vi "AnalogOutputs.vi"() -> ()   [LabVIEW 2016]
uses:
  controls/Enum.ctl
  <vilib>/rvi/errors/niLvFpgaAdjustHostInterfaceError.vi
  <vilib>/Utility/error.llb/Error Cluster From Error Code.vi
  controls/FPGAVIreferenceTypeDefScanEngine.ctl
  <vilib>/rvi/interface/nirviReadWriteControl/nirviReadWriteControl.xnode
  FPGA Bitfiles/lbniAFMControlle_scanControl_controllerFPGAPX_N4i+37z1gG8.lvbitx
  NiFpgaLv.dll
panel:
  in  "AO5.Activate":bool=TRUE
  in  "AO6.Activate":bool=TRUE
  in  "AO7.Activate":bool=TRUE
  in  "AO7":dbl(slide) caption="Bias" scale=-10.0..10.0
  in  "AO6":dbl(slide) caption="Bias" scale=-10.0..10.0
  in  "AO5":dbl(slide) caption="Bias" scale=-10.0..10.0
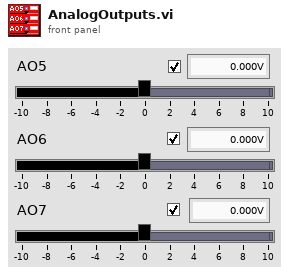
[diagram p1: front panel]
types:
  T1 = typedef "Enum.ctl" = enum16{"Init", "Read", "Write"}
  T2 = typedef "FPGAVIreferenceTypeDefScanEngine.ctl" = refnum<k20>
  T3 = enum8{"Enabled", "Disabled", "Disabled and Grayed Out"}
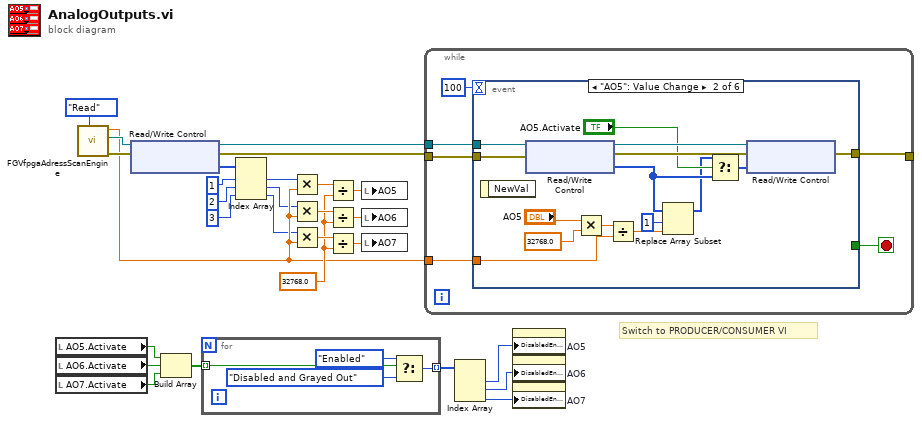
[diagram p0: block diagram]
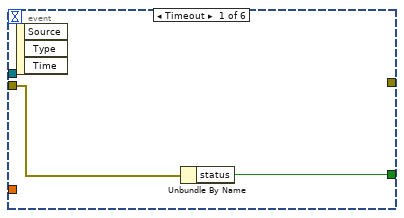
[diagram p2: hidden frame]
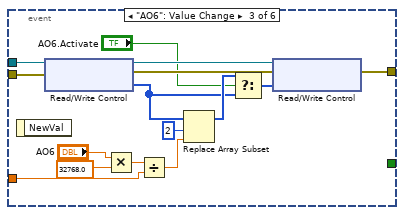
[diagram p3: hidden frame]
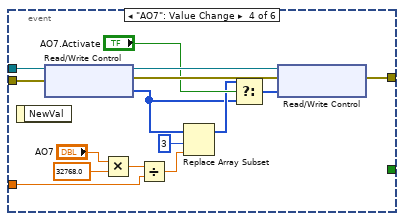
[diagram p4: hidden frame]
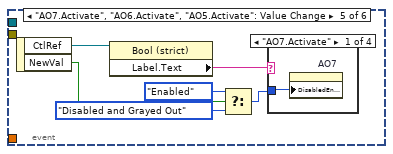
[diagram p5: hidden frame]
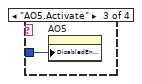
[diagram p7: hidden frame]
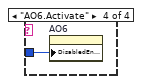
[diagram p8: hidden frame]
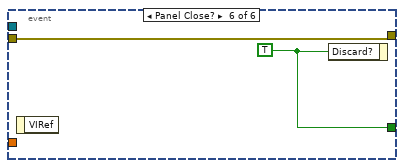
[diagram p9: hidden frame]
diagram:
  w5 = 32768.0 ("index")
  # "Switch to PRODUCER/CONSUMER VI"
  n1 = local read "AO5.Activate"() -> (w20:bool)
  n2 = local read "AO6.Activate"() -> (w19:bool)
  n3 = local read "AO7.Activate"() -> (w18:bool)
  n4 = call "FGVfpgaAdressScanEngine.vi"("Enum"=Enum."Read") -> ("error out"=w23:errorcluster, "FPGA.SEout"=w28:T2, "voltageRange(+/-)Out"=w4:dbl)  [unwired: 6 in, 2 out]
  n5 = xnode "Read/Write Control"("FPGA VI Reference In"=w28, "error in"=w23) -> ("FPGA VI Reference Out"=w10:T2, "error out"=w9:errorcluster, "aio.o.outputs"=w24:i16[])
  n6 = Build Array(w20, w19, w18) -> (w17:bool[])
  n7 = for {
    tunnel: w17 -> [w30] mode=indexing
    tunnel: [w29] -> w16 mode=indexing
    n8 = Select(t=T3."Enabled" ("Disabled"), s=w30, f=T3."Disabled and Grayed Out" ("Disabled")) -> (s? t:f=w29:T3)
  }
  n9 = Index Array(array=w24, index #1=1 ("index"), index #2=2 ("index"), index #3=3 ("index")) -> (element #1=w3:i16, element #2=w2:i16, element #3=w1:i16)
  n10 = Multiply(x=w3, y=w4) -> (x*y=w26:dbl)
  n11 = Multiply(x=w2, y=w4) -> (x*y=w22:dbl)
  n12 = Multiply(x=w1, y=w4) -> (x*y=w21:dbl)
  n13 = Divide(x=w26, y=w5) -> (x/y=w6:dbl)
  n14 = Divide(x=w22, y=w5) -> (x/y=w7:dbl)
  n15 = Divide(x=w21, y=w5) -> (x/y=w8:dbl)
  n16 = local write "AO5"(w6) -> ()
  n17 = local write "AO6"(w7) -> ()
  n18 = local write "AO7"(w8) -> ()
  n19 = while {
    tunnel: w4 -> [w35]
    tunnel: w9 -> [w33]
    tunnel: [w34] -> _
    tunnel: w10 -> [w36]
    stop <- w38 stop-if-true
    n20 = event shown="[1] \"AO5\": Value Change" {
      selector: _ -> [_ _ _ _ _ _]
      dyn-events: _ -> [_ _ _ _ _ _]
      timeout: 100 -> [_ _ _ _ _ _]
      tunnel: [w39 _ _ _ _ w96] -> w38
      tunnel: w36 -> [_ w48 w69 w83 _ _]
      tunnel: w35 -> [_ w46 w63 w78 _ _]
      tunnel: [_ w49 w66 w80 _ w95] -> w34
      tunnel: w33 -> [w40 w47 w67 w81 _ w95]
      event Timeout {
        n21 = event-data() -> ()  [unwired: 1 in, 3 out]
        n22 = Unbundle By Name(w40) -> ("status"=w39:bool)
      }
      event "AO5": Value Change {
        n23 = event-data() -> ()  [unwired: 1 in, 1 out]
        n24 = xnode "Read/Write Control"("FPGA VI Reference In"=w48, "error in"=w47) -> ("FPGA VI Reference Out"=w55:T2, "error out"=w50:errorcluster, "aio.o.outputs"=w43:i16[])
        n25 = Multiply(x="AO5", y=32768.0 ("index")) -> (x*y=w52:dbl)
        n26 = Divide(x=w52, y=w46) -> (x/y=w51:dbl)
        n27 = Replace Array Subset(array=w43, new element=w51, index=1) -> (w42:i16[])
        n28 = Select(t=w42, s="AO5.Activate", f=w43) -> (s? t:f=w41:i16[])
        n29 = xnode "Read/Write Control"("FPGA VI Reference In"=w55, "error in"=w50, "aio.o.outputs"=w41) -> ("error out"=w49:errorcluster)  [unwired: 1 out]
      }
      event "AO6": Value Change {
        n30 = event-data() -> ()  [unwired: 1 in, 1 out]
        n31 = xnode "Read/Write Control"("FPGA VI Reference In"=w69, "error in"=w67) -> ("FPGA VI Reference Out"=w68:T2, "error out"=w65:errorcluster, "aio.o.outputs"=w57:i16[])
        n32 = Multiply(x="AO6", y=32768.0 ("index")) -> (x*y=w60:dbl)
        n33 = Divide(x=w60, y=w63) -> (x/y=w64:dbl)
        n34 = Replace Array Subset(array=w57, new element=w64, index=2) -> (w59:i16[])
        n35 = Select(t=w59, s="AO6.Activate", f=w57) -> (s? t:f=w58:i16[])
        n36 = xnode "Read/Write Control"("FPGA VI Reference In"=w68, "error in"=w65, "aio.o.outputs"=w58) -> ("error out"=w66:errorcluster)  [unwired: 1 out]
      }
      event "AO7": Value Change {
        n37 = event-data() -> ()  [unwired: 1 in, 1 out]
        n38 = xnode "Read/Write Control"("FPGA VI Reference In"=w83, "error in"=w81) -> ("FPGA VI Reference Out"=w82:T2, "error out"=w85:errorcluster, "aio.o.outputs"=w72:i16[])
        n39 = Multiply(x="AO7", y=32768.0 ("index")) -> (x*y=w75:dbl)
        n40 = Divide(x=w75, y=w78) -> (x/y=w79:dbl)
        n41 = Replace Array Subset(array=w72, new element=w79, index=3) -> (w73:i16[])
        n42 = Select(t=w73, s="AO7.Activate", f=w72) -> (s? t:f=w71:i16[])
        n43 = xnode "Read/Write Control"("FPGA VI Reference In"=w82, "error in"=w85, "aio.o.outputs"=w71) -> ("error out"=w80:errorcluster)  [unwired: 1 out]
      }
      event "AO7.Activate", "AO6.Activate", "AO5.Activate": Value Change {
        n44 = event-data() -> ("CtlRef"=w91:refnum<vi>, "NewVal"=w89:bool)  [unwired: 1 in]
        n45 = property class="Bool (strict)"(reference=w91) -> ("Label.Text"=w90:string)  [unwired: 1 in, 2 out]
        n46 = Select(t=T3."Enabled" ("Disabled"), s=w89, f=T3."Disabled and Grayed Out" ("Disabled")) -> (s? t:f=w86:T3)
        n47 = case shown="\"AO7.Activate\"" w90 {
          tunnel: w86 -> [w92 _ w93 w94]
          frame "AO7.Activate" {
            n48 = property on="AO7" class="Slide (strict)"("DisabledEnum"=w92) -> ()  [unwired: 2 in, 2 out]
          }
          frame Default {
          }
          frame "AO5.Activate" {
            n49 = property on="AO5" class="Slide (strict)"("DisabledEnum"=w93) -> ()  [unwired: 2 in, 2 out]
          }
          frame "AO6.Activate" {
            n50 = property on="AO6" class="Slide (strict)"("DisabledEnum"=w94) -> ()  [unwired: 2 in, 2 out]
          }
        }
      }
      event Panel Close? {
        w96 = TRUE ("Discard?")
        n51 = event-data() -> ()  [unwired: 1 in, 1 out]
        n52 = event-data("Discard?"=w96) -> ()  [unwired: 1 in, 1 out]
      }
    }
  }
  n53 = Index Array(array=w16) -> (element #1=w15:T3, element #2=w14:T3, element #3=w13:T3)  [unwired: 3 in]
  n54 = property on="AO5" class="Slide (strict)"("DisabledEnum"=w15) -> ()  [unwired: 2 in, 2 out]
  n55 = property on="AO6" class="Slide (strict)"("DisabledEnum"=w14) -> ()  [unwired: 2 in, 2 out]
  n56 = property on="AO7" class="Slide (strict)"("DisabledEnum"=w13) -> ()  [unwired: 2 in, 2 out]
